vi "state machine.vi"() -> ()   [LabVIEW 2014]
uses:
  typedefs/state machine/performance data.ctl
  typedefs/test/test controls.ctl
panel:
  in  "Test Controls":T1 {"Lift" scale=-1.0..1.0; "Arm" scale=-1.0..1.0; "Drive Train Z" scale=0.0..10.0; "Drive Train Y" scale=-1.0..1.0; "Drive Train X" scale=-1.0..1.0}
  in  "Performance":T2
  # "Drive Encoders"
  # "Other Encoders"
  # "Pneumatics"
  # "Manual Override"
  # "Joystick Control"
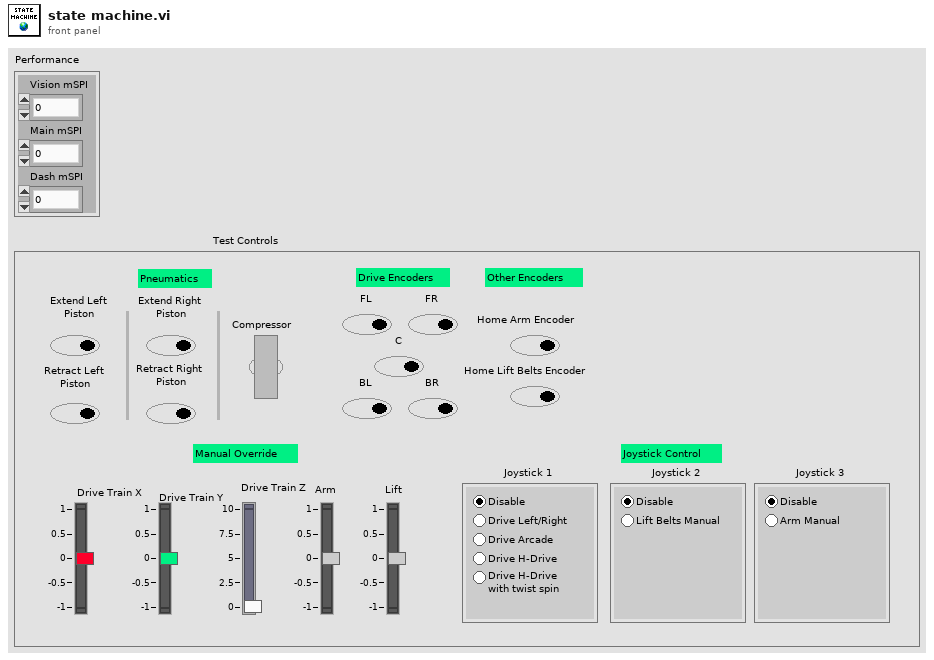
[diagram p1: front panel]
types:
  T1 = typedef "test controls.ctl" = cluster{"Drive Train X":dbl, "Drive Train Y":dbl, "Drive Train Z":dbl, "Extend Left \nPiston":bool, "Retract Left \nPiston":bool, "Extend Right \nPiston":bool, "Retract Right \nPiston":bool, "Compressor":bool, "Arm":dbl, "Lift":dbl, "FL":bool, "FR":bool, "BL":bool, "BR":bool, "C":bool, "Home Arm Encoder":bool, "Home Lift Belts Encoder":bool, "Joystick 1":enum32{"Disable", "Drive Left/Right", "Drive Arcade", "Drive H-Drive", "Drive H-Drive \nwith twist spin"}, "Joystick 2":enum32{"Disable", "Lift Belts Manual"}, "Joystick 3":enum32{"Disable", "Arm Manual"}}
  T2 = typedef "performance data.ctl" = cluster{"Vision mSPI":u32, "Main mSPI":u32, "Dash mSPI":u32}
diagram:
